vi "Sensors.vi"() -> ()   [LabVIEW 2013]
uses:
  <vilib>/Platform/TimedLoop/XDataNode/timing_clust.ctl
  <vilib>/Platform/TimedLoop/XDataNode/nitl_modes.ctl
  <vilib>/Platform/TimedLoop/XDataNode/wakeup.ctl
  <vilib>/Rock Robotics/SystemInterfaces/DIO/FPGA_DIOChannel.ctl
  <vilib>/Rock Robotics/SystemInterfaces/AI/FPGA_AIGyroChannel.ctl
  Program Files (x86)/National Instruments/LabVIEW 2013/examples/FRC/I2C/ADXL345 I2C/Driver/ADXL345 I2C Range.ctl
  Program Files (x86)/National Instruments/LabVIEW 2013/examples/FRC/I2C/ADXL345 I2C/Driver/ADXL345 I2C Axis.ctl
  <vilib>/Rock Robotics/WPI/Counter/WPI_CounterDigitalInputToDigitalSource.vi
  <vilib>/Platform/TimedLoop/XDataNode/XDataNode.xnode
  <vilib>/Platform/TimedLoop/XDataNode/XDNodeRunTimeDep.lvlib
panel:
  out "Direction":dbl(knob)
  out "Velocity":dbl
  out "Battery Voltage":dbl
  out "Acceleration":dbl
  out "Pantograph":i16[](graph)
  in  "Wheel diameter":dbl=1.0
  out "Current angle":dbl
  out "Distance":dbl
  out "Revolutions":dbl
  in  "Reset Gyro":bool
  in  "Reset Encoder":bool
  out "Encoder Rate":dbl
  out "Gyro":dbl(knob)
  in  "stop":bool
  # "Drive Motors"
  # "Encoder"
  # "Motion"
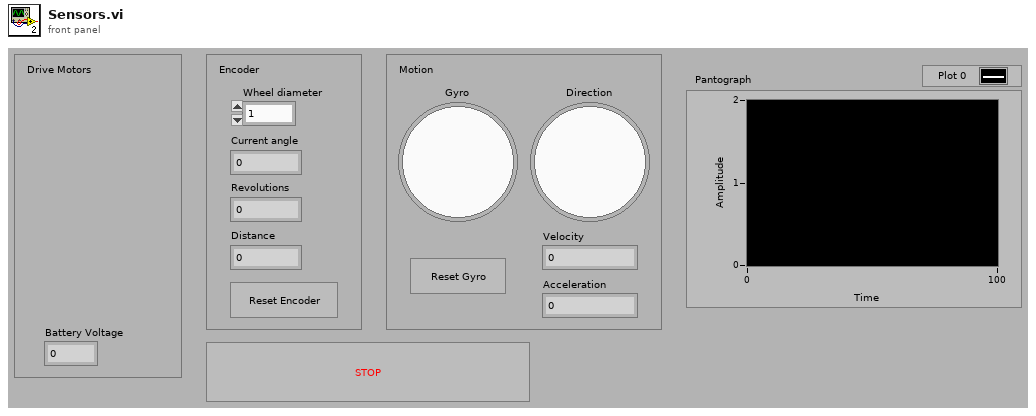
[diagram p1: front panel]
types:
  T1 = typedef "ADXL345 I2C Range.ctl" = u8
  T2 = typedef "FPGA_AIGyroChannel.ctl" = enum8{"AI 1", "AI 2", "Invalid"}
  T3 = typedef "FPGA_DIOChannel.ctl" = enum8{"DIO 1", "DIO 2", "DIO 3", "DIO 4", "DIO 5", "DIO 6", "DIO 7", "DIO 8", "DIO 9", "DIO 10", "DIO 11", "DIO 12", "DIO 13", "DIO 14", "Invalid"}
  T4 = typedef "WPI_DigitalInputDevRef.ctl" = cluster{"DevStatus":errorcluster, "DIO Channel":T3, "Digital Module":T5}
  T5 = typedef "FPGA_TypedefDigitalModule.ctl" = enum16{"Digital Module 1", "Digital Module 2"}
  T6 = typedef "WPI_GyroDevRef.ctl" = cluster{"DevStatus":errorcluster, "Analog Module":T7, "Analog Channel":T8, "Offset":dbl, "Gain (VoltsPerDegree/Second)":dbl}
  T7 = typedef "FPGA_TypedefAnalogModule.ctl" = enum16{"Analog Module 1", "Analog Module 2"}
  T8 = typedef "FPGA_AIChannel.ctl" = enum8{"AI 1", "AI 2", "AI 3", "AI 4", "AI 5", "AI 6", "AI 7", "AI 8", "Invalid"}
  T9 = typedef "FPGA_CounterEncoderSourceConvertionLVSourceType.ctl" = cluster{"DevStatus":errorcluster, "AnalogTriggerMode?":bool, "DigitalMode":cluster{"Digital Module":T5, "DIO Channel":T10}, "AnalogTriggerMode":cluster{"AnalogTriggerIndex":T11, "OutputType":T12}}
  T10 = typedef "FPGA_DIODigitalSourceChannel.ctl" = enum8{"DIO 1", "DIO 2", "DIO 3", "DIO 4", "DIO 5", "DIO 6", "DIO 7", "DIO 8", "DIO 9", "DIO 10", "DIO 11", "DIO 12", "DIO 13", "DIO 14", "Disabled"}
  T11 = typedef "FPGA_AnalogTriggerIndex.ctl" = enum8{"Trig 0", "Trig 1", "Trig 2", "Trig 3", "Trig 4", "Trig 5", "Trig 6", "Trig 7", "Invalid"}
  T12 = typedef "FPGA_AnalogTriggerOutType.ctl" = enum16{"InWindow", "TriggerState", "Rising", "Falling"}
  T13 = typedef "WPI_EncoderDevRef.ctl" = cluster{"DevStatus":errorcluster, "EncoderIndex":T14, "CounterIndex":T15, "DistancePerCount":dbl, "Decoding Type":T16}
  T14 = typedef "FPGA_EncoderIdx.ctl" = enum8{"Enc 0", "Enc 1", "Enc 2", "Enc 3", "Invalid"}
  T15 = typedef "FPGA_CounterCtrSystemIndex.ctl" = enum8{"Ctr 0", "Ctr 1", "Ctr 2", "Ctr 3", "Ctr 4", "Ctr 5", "Ctr 6", "Ctr 7", "Invalid"}
  T16 = typedef "WPI_EncoderType.ctl" = enum16{"1x", "2x", "4x"}
  T17 = typedef "XDNodeRunTimeDep.lvlib/timing_clust.ctl" = cluster{"Expected End [f-1]":u64, "Actual End [f-1]":u64, "Finished Late? [f-1]":bool, "Expected End [i-1]":u64, "Actual End [i-1]":u64, "Finished Late? [i-1]":bool, "Expected Start [i]":u64, "Actual Start [i]":u64, "Expected Start [f]":u64, "Actual Start [f]":u64, "Source Name":string, "Structure Name":string, "Period":i64, "Deadline":i64, "Offset":i64, "Start":i64, "Priority":i32, "Timeout":i32, "Mode":T18, "Wakeup Reason":T19, "Error":errorcluster, "Source Type":string, "Secondary Source Type":string, "Global End Time":u64, "Global Start Time":u64, "Frame Duration":u64, "Iteration Duration":u64, "Assigned CPU":i32, "I/O Scan Engine Mode":u32}
  T18 = typedef "XDNodeRunTimeDep.lvlib/nitl_modes.ctl" = enum32{"No Change", "Process missed periods, maintain original phase", "Discard missed periods, maintain original phase", "Process missed periods, ignore original phase", "Discard missed periods, ignore original phase"}
  T19 = typedef "XDNodeRunTimeDep.lvlib/wakeup.ctl" = enum32{"Normal", "Aborted", "Asynchronous wakeup", "Timing source error", "Timed loop error", "Timeout"}
  T20 = typedef "WPI_I2CDevRef.ctl" = cluster{"DevStatus":errorcluster, "Digital Module":T5, "Device Address":u8}
  T21 = typedef "ADXL345 I2C Axis.ctl" = u8
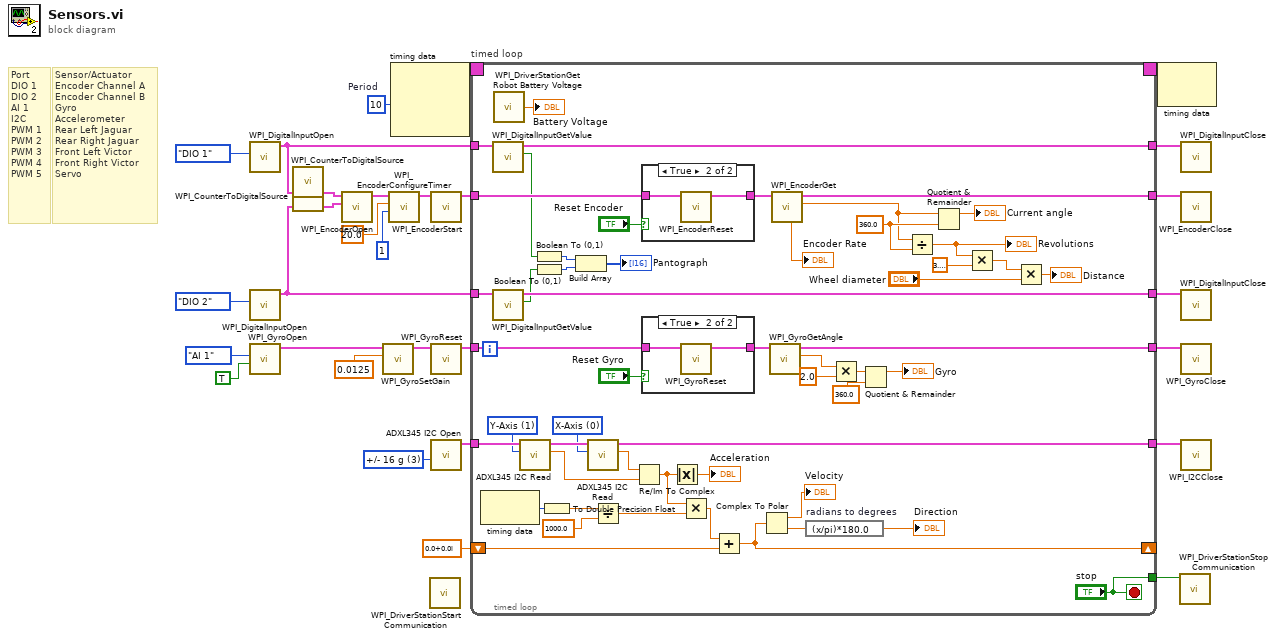
[diagram p0: block diagram]
diagram:
  w6 = T1 3 items=["+/- 2 g", "+/- 4 g", "+/- 8 g", "+/- 16 g"] ("Range")
  w27 = i64 10  # Period
  # "Sensor/Actuator\nEncoder Channel A\nEncoder Channel B\nGyro\nAccelerometer\nRear Left Jaguar\nRear Right Jaguar\nFront Left Victor\nFront Right Victor\nServo"
  # "Port\nDIO 1\nDIO 2\nAI 1\nI2C\nPWM 1\nPWM 2\nPWM 3\nPWM 4\nPWM 5"
  n1 = call <vilib>:"WPI_DigitalInputOpen.vi"("DIO Channel"=FPGA_DIOChannel."DIO 1") -> ("DigitalInputDevRef"=w19:T4)  [unwired: 9 in, 1 out]
  n2 = call <vilib>:"WPI_DigitalInputOpen.vi"("DIO Channel"=FPGA_DIOChannel."DIO 2") -> ("DigitalInputDevRef"=w20:T4)  [unwired: 9 in, 1 out]
  n3 = call <vilib>:"WPI_GyroOpen.vi"("Calibrate On Open"=TRUE, "Analog Channel"=FPGA_AIGyroChannel."AI 1") -> ("GyroDevRef"=w12:T6)  [unwired: 7 in, 2 out]
  n4 = call-poly <vilib>:"WPI_CounterToDigitalSource.vi"("DigitalInputDevRef"=w19) -> ("Digital Source"=w22:T9)  [unwired: 6 in]
  n5 = call-poly <vilib>:"WPI_CounterToDigitalSource.vi"("DigitalInputDevRef"=w20) -> ("Digital Source"=w21:T9)  [unwired: 6 in]
  n6 = call <vilib>:"WPI_EncoderOpen.vi"("BSource"=w21, "ASource"=w22) -> ("EncoderDevRef"=w10:T13)  [unwired: 8 in, 1 out]
  n7 = call <vilib>:"WPI_GyroSetGain.vi"("Gain (VoltsPerDegree/Second)"=0.0125, "GyroDevRef"=w12) -> ("GyroDevRef"=w3:T6)  [unwired: 1 in, 8 out]
  n8 = call <vilib>:"WPI_EncoderConfigureTimer.vi"("Number Samples to Average"=u8 1, "Minimum Rate"=20.0, "EncoderDevRef"=w10) -> ("EncoderDevRef"=w9:T13)  [unwired: 1 in, 7 out]
  n9 = node-c288(w27) -> (w29:T17)  [unwired: 2 out]
  n10 = call <vilib>:"WPI_DriverStationStart Communication.vi"() -> ()  [unwired: 1 in, 11 out]
  n11 = call <vilib>:"WPI_EncoderStart.vi"("EncoderDevRef"=w9) -> ("EncoderDevRef"=w15:T13)  [unwired: 9 in, 1 out]
  n12 = call <vilib>:"WPI_GyroReset.vi"("GyroDevRef"=w3) -> ("GyroDevRef"=w2:T6)  [unwired: 9 in, 1 out]
  n13 = call "ADXL345 I2C Open.vi"("Range"=w6) -> ("I2CDevRef"=w5:T20)  [unwired: 3 in, 7 out]
  n14 = timed-loop "timed loop" {
    timing: w29 -> [_]
    timing-out: [_] -> w28
    tunnel: [w81] -> _
    tunnel: w19 -> [w81]
    tunnel: w20 -> [w80]
    tunnel: [w77] -> w16
    tunnel: [w59] -> w17
    tunnel: w2 -> [w69]
    tunnel: [w76] -> w23
    tunnel: w15 -> [w74]
    tunnel: [w61] -> w18
    tunnel: ["stop"] -> w14
    tunnel: [w47] -> w4
    tunnel: w5 -> [w32]
    shift-right: [w36] -> _
    shift-left: cdb 0.0+0.0i ("x") -> [w37]
    stop <- "stop" stop-if-true
    w52 = T21 0 items=["X-Axis", "Y-Axis", "Z-Axis"] ("Axis")
    w31 = T21 1 items=["X-Axis", "Y-Axis", "Z-Axis"] ("Axis")
    w67 = 360.0 ("y")
    n15 = node-c288() -> (w34:i64)  [unwired: 1 out]
    n16 = call <vilib>:"WPI_DigitalInputGetValue.vi"("DigitalInputDevRef"=w81) -> ("Value"=w71:bool, "DigitalInputDevRef"=w59:T4)  [unwired: 8 in, 1 out]
    n17 = call <vilib>:"WPI_DigitalInputGetValue.vi"("DigitalInputDevRef"=w80) -> ("Value"=w58:bool, "DigitalInputDevRef"=w77:T4)  [unwired: 8 in, 1 out]
    n18 = call <vilib>:"WPI_DriverStationGet Robot Battery Voltage.vi"() -> ("robot battery voltage"=→"Battery Voltage":dbl)  [unwired: 14 in, 1 out]
    n19 = call "ADXL345 I2C Read.vi"("Axis"=w31, "I2CDevRef"=w32) -> ("Acceleration"=w41:dbl, "I2CDevRef Out"=w53:T20)  [unwired: 1 in, 7 out]
    n20 = Boolean To (0,1)(Boolean=w71) -> (0, 1=w79:i16)
    n21 = Boolean To (0,1)(Boolean=w58) -> (0, 1=w78:i16)
    n22 = To Double Precision Float(number=w34) -> (double precision float=w46:dbl)
    n23 = Build Array(w79, w78) -> (→"Pantograph":i16[])
    n24 = call "ADXL345 I2C Read.vi"("Axis"=w52, "I2CDevRef"=w53) -> ("Acceleration"=w42:dbl, "I2CDevRef Out"=w47:T20)  [unwired: 1 in, 7 out]
    n25 = Divide(x=w46, y=1000.0) -> (x/y=w44:dbl)
    n26 = Re/Im To Complex(1:w41, 2:w42) -> (0:w30:cdb)
    n27 = case shown="True" "Reset Encoder" {
      tunnel: w74 -> [w87 w89]
      tunnel: [w87 w88] -> w73
      frame False {
      }
      frame True {
        n28 = call <vilib>:"WPI_EncoderReset.vi"("EncoderDevRef"=w89) -> ("EncoderDevRef"=w88:T13)  [unwired: 1 in, 9 out]
      }
    }
    n29 = case shown="True" "Reset Gyro" {
      tunnel: w69 -> [w84 w86]
      tunnel: [w84 w85] -> w68
      frame False {
      }
      frame True {
        n30 = call <vilib>:"WPI_GyroReset.vi"("GyroDevRef"=w86) -> ("GyroDevRef"=w85:T6)  [unwired: 9 in, 1 out]
      }
    }
    n31 = Absolute Value(x=w30) -> (abs(x)=→"Acceleration":dbl)
    n32 = Multiply(x=w30, y=w44) -> (x*y=w38:cdb)
    n33 = Add(x=w38, y=w37) -> (x+y=w36:cdb)
    n34 = Complex To Polar(r * e^(i*theta)=w36) -> (r=→"Velocity":dbl, theta=w39:dbl)
    n35 = call <vilib>:"WPI_GyroGetAngle.vi"("GyroDevRef"=w68) -> ("Angle"=w55:dbl, "GyroDevRef"=w76:T6)  [unwired: 7 in, 2 out]
    n36 = call <vilib>:"WPI_EncoderGet.vi"("EncoderDevRef"=w73) -> ("Distance"=w60:dbl, "EncoderDevRef"=w61:T13, "Rate"=→"Encoder Rate":dbl)  [unwired: 5 in, 3 out]
    n37 = expression code="(x/pi)*180.0" "radians to degrees"(w39) -> (→"Direction":dbl)
    n38 = Multiply(x=w55, y=2.0) -> (x*y=w50:dbl)
    n39 = Quotient & Remainder(x=w50, y=360.0) -> (x-y*floor(x/y)=→"Gyro":dbl)  [unwired: 1 out]
    n40 = Divide(x=w60, y=w67) -> (x/y=w66:dbl)
    "Revolutions" <- w66
    n41 = Quotient & Remainder(x=w60, y=w67) -> (x-y*floor(x/y)=→"Current angle":dbl)  [unwired: 1 out]
    n42 = Multiply(x=w66, y=3.141592653589793) -> (x*y=w63:dbl)
    n43 = Multiply(x=w63, y="Wheel diameter") -> (x*y=→"Distance":dbl)
  }
  n44 = node-c288(w28) -> ()  [unwired: 1 out]
  n45 = call <vilib>:"WPI_DriverStationStop Communication.vi"("StopCommunication"=w14) -> ()  [unwired: 1 in, 10 out]
  n46 = call <vilib>:"WPI_DigitalInputClose.vi"("DigitalInputDevRef"=w17) -> ()  [unwired: 10 in, 1 out]
  n47 = call <vilib>:"WPI_EncoderClose.vi"("EncoderDevRef"=w18) -> ()  [unwired: 10 in, 1 out]
  n48 = call <vilib>:"WPI_DigitalInputClose.vi"("DigitalInputDevRef"=w16) -> ()  [unwired: 10 in, 1 out]
  n49 = call <vilib>:"WPI_GyroClose.vi"("GyroDevRef"=w23) -> ()  [unwired: 10 in, 1 out]
  n50 = call <vilib>:"WPI_I2CClose.vi"("I2CDevRef"=w4) -> ()  [unwired: 10 in, 1 out]
